vi "Test Progess Bar.vi"() -> ()   [LabVIEW 2015]
uses:
  Progress Bar Cluster.ctl
  Progress Bar Action.ctl
panel:
  in  "stop":bool
  in  "Send":bool
  in  "element":T1
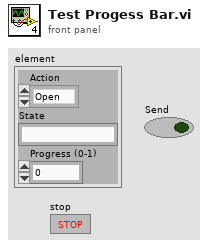
[diagram p1: front panel]
types:
  T1 = typedef "Progress Bar Cluster.ctl" = cluster{"Action":T2, "State":string, "Progress (0-1)":dbl}
  T2 = typedef "Progress Bar Action.ctl" = enum16{"Open", "Update", "Close", "End"}
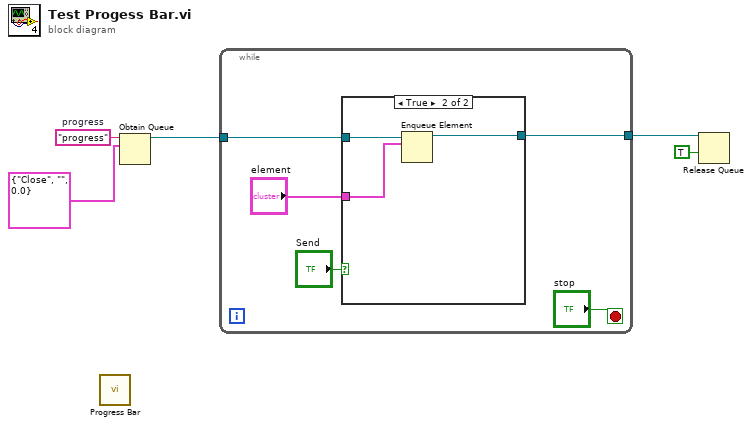
[diagram p0: block diagram]
diagram:
  w5 = "progress"  # progress
  n1 = call "Progress Bar.vi"() -> ()  [unwired: 12 in]
  n2 = Obtain Queue(name (unnamed)=w5, element data type=T1 {"Action"=enum."Close", "State"="", "Progress (0-1)"=0.0}) -> (queue out=w3:refnum<queue>)  [unwired: 3 in, 2 out]
  n3 = while {
    tunnel: w3 -> [w10]
    tunnel: [w6] -> w2
    stop <- "stop" stop-if-true
    n4 = case shown="True" "Send" {
      tunnel: w10 -> [w11 w14]
      tunnel: "element" -> [_ w13]
      tunnel: [w11 w12] -> w6
      frame False {
      }
      frame True {
        n5 = Enqueue Element(queue=w14, element=w13) -> (queue out=w12:refnum<queue>)  [unwired: 2 in, 2 out]
      }
    }
  }
  n6 = Release Queue(queue=w2, force destroy? (F)=TRUE) -> ()  [unwired: 1 in, 3 out]
